vi "Hatch Extend Controller.vi"(8 "error in":errorcluster) -> ()   [LabVIEW 2019]
doc: "This VI executes continuously carrying out the current operation and responding to updates or new operations. It will often contain the timing or control code that is difficult to place directly in TeleOp. This VI generally opens all sensors and motors and isolates the rest of the robot code from knowing how the operations are carried out."
uses:
  <vilib>/Rock Robotics/WPI/Framework/Completion Status.ctl
  Hatch Extend Setpoints.ctl
  Hatch Extend Operations.ctl
  <vilib>/Rock Robotics/WPI/SafetyOutput/WPI_SafetyOutputConfigMenu.ctl
  <vilib>/Rock Robotics/Network Tables/NT Write Boolean.vi
panel:
  in  "Interactive Values":T1
  out "Current\nCmd":string
  in  "Buttons":cluster{"Execute Cmd":bool, "Abort Cmd":bool}
  out "Command Timing":cluster{"Start Time (ms)":u32, "Iterations":i32}
  out "Status":T3
  # "Tip: It may be helpful to observe inputs and sensor values.\nYou may also want to display tuning or debugging controls."
  # "Interactive Command: You may fill in the settings for a command\nand schedule it with the Execute button. You can observe and abort\nany command while fine tuning the code for the controller."
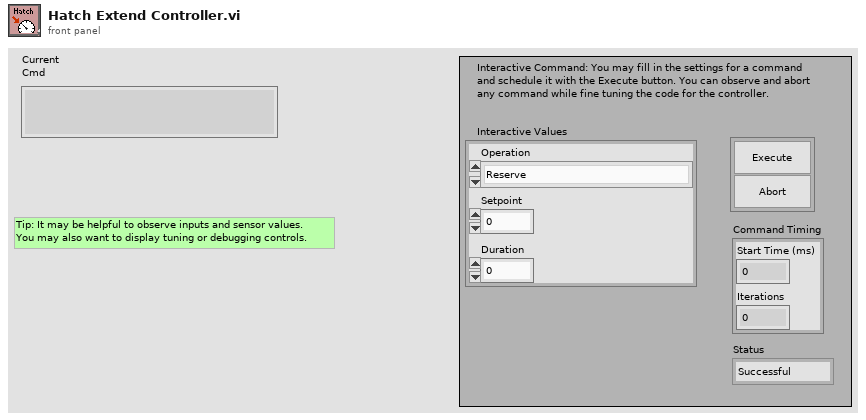
[diagram p1: front panel]
types:
  T1 = typedef "Hatch Extend Setpoints.ctl" = cluster{"Operation":T2, "Setpoint":dbl, "Duration":dbl}
  T2 = typedef "Hatch Extend Operations.ctl" = enum16{"Reserve", "Read Current", "Immediate", "Extend", "Retract"}
  T3 = typedef "Completion Status.ctl" = enum16{"Successful", "Aborted", "Incomplete"}
  T4 = typedef "WPI_SafetyOutputConfigMenu.ctl" = enum16{"Enable", "Disable"}
  T5 = typedef "WPI_MotorControlDeviceRef.ctl" = cluster{"DeviceStatus":errorcluster, "Type":T6, "PWM":cluster{"PWM Channel":T7, "DeadBand":T8}, "CAN":cluster{"Device Number":u8, "SetOutput VI Ref":variant, "GetOutput VI Ref":variant, "Enable VI Ref":variant, "Disable VI Ref":variant, "Data":variant}, "Invert":bool, "DIO PWM":cluster{"PWM \"Enable\" Channel":T7, "DIOChannel":T9, "PWM Rate":dbl}}
  T6 = typedef "WPI_MotorControlType.ctl" = enum16{"PWM", "CAN", "DIO PWM"}
  T7 = typedef "FPGA_DIOPWMChannel.ctl" = enum8{"PWM 0", "PWM 1", "PWM 2", "PWM 3", "PWM 4", "PWM 5", "PWM 6", "PWM 7", "PWM 8", "PWM 9", "PWM MXP 0", "PWM MXP 1", "PWM MXP 2", "PWM MXP 3", "PWM MXP 4", "PWM MXP 5", "PWM MXP 6", "PWM MXP 7", "PWM MXP 8", "PWM MXP 9", "Invalid"}
  T8 = typedef "WPI_PWMDeadband.ctl" = cluster{"Name":string, "maxPositivePwm":i32, "minPositivePwm":i32, "centerPwm":i32, "maxNegativePwm":i32, "minNegativePwm":i32, "angularRange":u16}
  T9 = typedef "FPGA_DIOChannel.ctl" = enum8{"DIO 0", "DIO 1", "DIO 2", "DIO 3", "DIO 4", "DIO 5", "DIO 6", "DIO 7", "DIO 8", "DIO 9", "DIO MXP 0", "DIO MXP 1", "DIO MXP 2", "DIO MXP 3", "DIO MXP 4", "DIO MXP 5", "DIO MXP 6", "DIO MXP 7", "DIO MXP 8", "DIO MXP 9", "DIO MXP 10", "DIO MXP 11", "DIO MXP 12", "DIO MXP 13", "DIO MXP 14", "DIO MXP 15", "SPI Port CS1", "SPI Port CS2", "SPI Port CS3", "SPI Port MISO", "SPI Port MOSI", "Invalid"}
  T10 = typedef "Command Status Info.ctl" = cluster{"Name":string, "Status":T3, "notifier out":T11}
  T11 = typedef "Completion Notifier.ctl" = refnum<notifier>
  T12 = cluster{"Current Command":T1, "Command Timing":cluster{"Start Time (ms)":u32, "Iterations":i32}, "Command Arguments":cluster{"Command Info":T10, "Description":string, "Default Command":T1, "queue out":refnum<queue>, "Subsystem Name":string}}
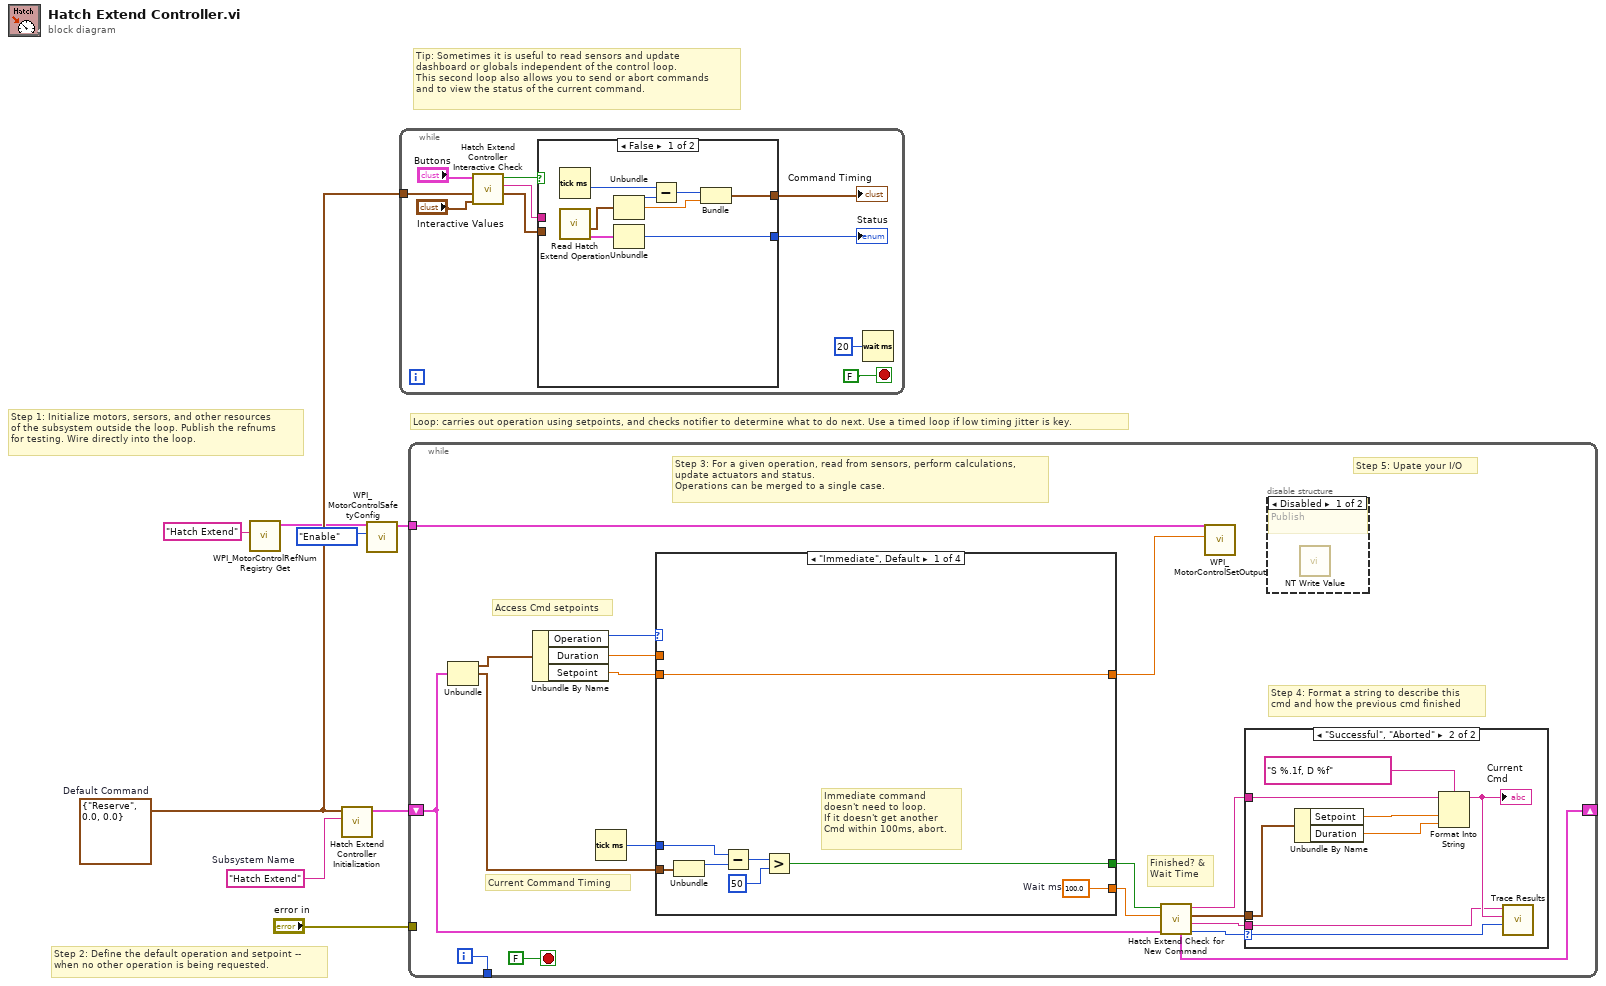
[diagram p0: block diagram]
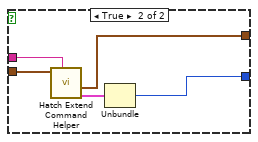
[diagram p2: hidden frame]
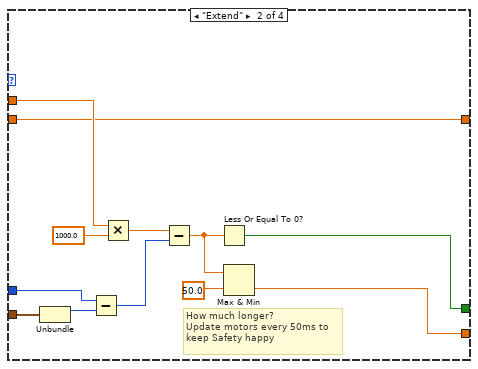
[diagram p5: hidden frame]
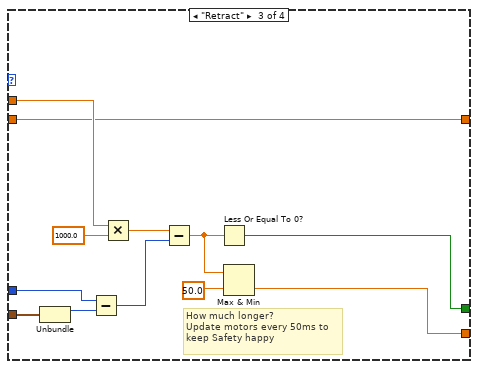
[diagram p6: hidden frame]
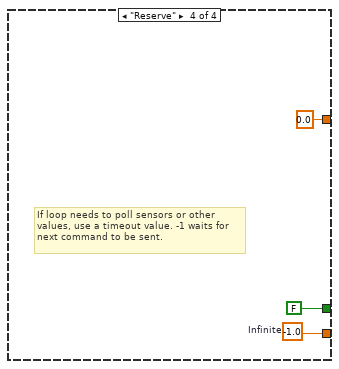
[diagram p7: hidden frame]
diagram:
  w5 = T1 {"Operation"=enum."Reserve", "Setpoint"=0.0, "Duration"=0.0}  # Default Command
  w6 = "Hatch Extend"  # Subsystem Name
  # "Tip: Sometimes it is useful to read sensors and update\ndashboard or globals independent of the control loop.\nThis second loop also allows you to send or abort commands\nand to view the status of the current command."
  # "Step 2: Define the default operation and setpoint --\nwhen no other operation is being requested."
  # "Step 1: Initialize motors, sersors, and other resources\nof the subsystem outside the loop. Publish the refnums\nfor testing. Wire directly into the loop."
  # "Loop: carries out operation using setpoints, and checks notifier to determine what to do next. Use a timed loop if low timing jitter is key."
  n1 = call <vilib>:"WPI_MotorControlRefNum Registry Get.vi"("refnum name"="Hatch Extend") -> ("MotorControlDevRef"=w3:T5)  [unwired: 9 in, 1 out]
  n2 = call "Hatch Extend Controller Initialization.vi"("Subsystem Name"=w6, "Default Command"=w5) -> ("Current Command"=w7:T12)  [unwired: 9 in]
  n3 = call <vilib>:"WPI_MotorControlSafetyConfig.vi"("mode"=WPI_SafetyOutputConfigMenu."Enable", "MotorControlDevRef"=w3) -> ("MotorControlDevRef"=w1:T5)  [unwired: 8 in, 1 out]
  n4 = while {
    tunnel: w5 -> [w15]
    stop <- FALSE stop-if-true
    n5 = call "Hatch Extend Controller Interactive Check.vi"("Interactive Command in"="Interactive Values", "Default Command"=w15, "Buttons"="Buttons") -> ("Interactive Command out"=w12:T1, "Trace String"=w13:string, "Schedule"=w14:bool)  [unwired: 6 in]
    n6 = case shown="False" w14 {
      tunnel: [w26 w31] -> w11
      tunnel: w12 -> [_ w29]
      tunnel: [w22 w27] -> w10
      tunnel: w13 -> [_ w30]
      frame False {
        n7 = Tick Count (ms)() -> (millisecond timer value=w21:u32)
        n8 = call "Read Hatch Extend Operation.vi"() -> ("Command Info"=w19:T10, "SubSystem Data"=w20:T1)  [unwired: 9 in, 1 out]
        n9 = Unbundle(w20) -> ("Operation"=w25:T2, "Setpoint"=w23:dbl)  [unwired: 1 out]
        n10 = Unbundle(w19) -> ("Status"=w26:T3)  [unwired: 2 out]
        n11 = Subtract(x=w21, y=w25) -> (x-y=w24:u32)
        n12 = Bundle(w24, "Setpoint"=w23) -> (w22:cluster{u32, "Setpoint":dbl})  [unwired: 1 in]
      }
      frame True {
        n13 = call "Hatch Extend Command Helper.vi"("Description"=w30, "SubSystem Data"=w29) -> ("Command Info Out"=w28:T10, "Command Timing"=w27:cluster{"Start Time (ms)":u32, "Iterations":i32})  [unwired: 7 in, 1 out]
        n14 = Unbundle(w28) -> ("Status"=w31:T3)  [unwired: 2 out]
      }
    }
    "Status" <- w11
    "Command Timing" <- w10
    n15 = Wait (ms)(milliseconds to wait=u32 20) -> ()  [unwired: 1 out]
  }
  n16 = while {
    shift-right: [w41] -> _
    shift-left: w7 -> [w34]
    tunnel: [w48] -> _
    tunnel: "error in" -> [_]
    tunnel: w1 -> [w33]
    i -> [w48]
    stop <- FALSE stop-if-true
    # "Step 5: Upate your I/O"
    # "Step 4: Format a string to describe this\ncmd and how the previous cmd finished"
    # "Current Command Timing"
    # "Access Cmd setpoints"
    # "Finished? &\nWait Time"
    # "Step 3: For a given operation, read from sensors, perform calculations,\nupdate actuators and status.\nOperations can be merged to a single case."
    n17 = Unbundle(w34) -> ("Current Command"=w47:T1, "Command Timing"=w43:cluster{"Start Time (ms)":u32, "Iterations":i32})  [unwired: 1 out]
    n18 = Unbundle By Name(w47) -> ("Operation"=w46:T2, "Duration"=w45:dbl, "Setpoint"=w42:dbl)
    n19 = Tick Count (ms)() -> (millisecond timer value=w44:u32)
    n20 = case shown="\"Immediate\", Default" w46 {
      tunnel: [w65 w67 w79 w92] -> w39
      tunnel: [w59 w66 w78 FALSE ("ignore previous (F)")] -> w40
      tunnel: w43 -> [w61 w70 w82 _]
      tunnel: w45 -> [_ w69 w81 _]
      tunnel: w44 -> [w60 w71 w83 _]
      tunnel: w42 -> [w58 w68 w80 _]
      tunnel: [w58 w68 w80 0.0 ("Setpoint")] -> w32
      frame "Immediate", Default {
        w65 = 100.0  # Wait ms
        # "Immediate command\ndoesn't need to loop.\nIf it doesn't get another\nCmd within 100ms, abort."
        n21 = Unbundle(w61) -> ("Start Time (ms)"=w64:u32)  [unwired: 1 out]
        n22 = Subtract(x=w60, y=w64) -> (x-y=w63:u32)
        n23 = Greater?(x=w63, y=u8 50 ("Left Motor")) -> (0:w59:bool)
      }
      frame "Extend" {
        # "How much longer?\nUpdate motors every 50ms to\nkeep Safety happy"
        n24 = Unbundle(w70) -> ("Start Time (ms)"=w74:u32)  [unwired: 1 out]
        n25 = Subtract(x=w71, y=w74) -> (x-y=w77:u32)
        n26 = Multiply(x=w69, y=1000.0) -> (x*y=w76:dbl)
        n27 = Subtract(x=w76, y=w77) -> (x-y=w73:dbl)
        n28 = Less Or Equal To 0?(x=w73) -> (x <= 0?=w66:bool)
        n29 = Max & Min(x=w73, y=50.0) -> (min(x,y)=w67:dbl)  [unwired: 1 out]
      }
      frame "Retract" {
        # "How much longer?\nUpdate motors every 50ms to\nkeep Safety happy"
        n30 = Unbundle(w82) -> ("Start Time (ms)"=w86:u32)  [unwired: 1 out]
        n31 = Subtract(x=w83, y=w86) -> (x-y=w89:u32)
        n32 = Multiply(x=w81, y=1000.0) -> (x*y=w88:dbl)
        n33 = Subtract(x=w88, y=w89) -> (x-y=w85:dbl)
        n34 = Less Or Equal To 0?(x=w85) -> (x <= 0?=w78:bool)
        n35 = Max & Min(x=w85, y=50.0) -> (min(x,y)=w79:dbl)  [unwired: 1 out]
      }
      frame "Reserve" {
        w92 = -1.0  # Infinite
        # "If loop needs to poll sensors or other\nvalues, use a timeout value. -1 waits for\nnext command to be sent."
      }
    }
    n36 = call "Hatch Extend Check for New Command.vi"("Current Command"=w34, "Wait time (ms)"=w39, "Finished?"=w40) -> ("Completion"=w35:T3, "Subsystem Name"=w36:string, "Current Command"=w37:T1, "Initial Trace String"=w38:string, "NextCommand"=w41:T12)  [unwired: 4 in]
    n37 = call <vilib>:"WPI_MotorControlSetOutput.vi"("Output"=w32, "MotorControlDevRef"=w33) -> ()  [unwired: 7 in, 3 out]
    n38 = case shown="\"Successful\", \"Aborted\"" w35 {
      selector: w35 -> [_ w57]
      tunnel: w38 -> [_ w53]
      tunnel: w37 -> [_ w54]
      tunnel: w36 -> [_ w50]
      frame "Incomplete", Default {
        # "Continuing current command"
      }
      frame "Successful", "Aborted" {
        # "Report and setup for next command"
        n39 = Unbundle By Name(w54) -> ("Setpoint"=w56:dbl, "Duration"=w51:dbl)
        n40 = Format Into String(format string="S %.1f, D %f", initial string=w53, w56, w51) -> (resulting string=w52:string)  [unwired: 1 in, 1 out]
        "Current\nCmd" <- w52
        n41 = call <vilib>:"Trace Results.vi"("Status of previous command"=w57, "Description"=w52, "Subsystem"=w50) -> ()  [unwired: 9 in]
      }
    }
    n42 = disable-structure shown="Disabled" {
      frame Disabled {
        # "Publish"
        n43 = call-poly <vilib>:"NT Write Value.vi"() -> ()  [unwired: 11 in, 1 out]
      }
      frame Enabled {
      }
    }
  }
